vi "Exp2.vi"() -> ()   [LabVIEW 2018]
uses:
  <vilib>/Platform/TimedLoop/XDataNode/timing_clust.ctl
  <vilib>/Platform/TimedLoop/XDataNode/nitl_modes.ctl
  <vilib>/Platform/TimedLoop/XDataNode/wakeup.ctl
  <vilib>/MakerHub/LINX/Public/Peripherals/Analog/Analog Read 1 Chan.vi
  <vilib>/MakerHub/LINX/Public/Peripherals/PWM/PWM Set Duty Cycle 1 Chan.vi
  <vilib>/MakerHub/LINX/Public/Peripherals/Analog/Analog Read N Chans.vi
  <vilib>/MakerHub/LINX/Private/Local IO/LinxAnalogRead.vi
  <vilib>/MakerHub/LINX/Public/Utilities/Check Channel.vi
  <vilib>/MakerHub/LINX/Public/Utilities/Open Serial.vi
  <vilib>/MakerHub/LINX/Private/Utilties/Generate Error.vi
  <vilib>/MakerHub/LINX/Public/Peripherals/PWM/PWM Set Duty Cycle N Chans.vi
  <vilib>/platform/TimedLoop/XDataNode/XDataNode.xnode
  <vilib>/MakerHub/LINX/LMH-LINX.lvlib
  <vilib>/Platform/TimedLoop/XDataNode/XDNodeRunTimeDep.lvlib
panel:
  out "T0":dbl
  in  "Tab Control":enum32{"Monitoring", "TDTC Model"}(tab)
  out "Temperature":cluster{dbl, "output":dbl}(graph)={31.0, "output"=73.73046875}
  out "Overrun":bool
  in  "Serial Port":refnum<visa-resource-name>="COM4"
  in  "Duty Cycle (0-100)":dbl min=0.0 max=1.0 step=0.1
  out "Period":i64
  in  "Kss":dbl=1.1
  in  "Theta":dbl=9.49
  in  "Tau":dbl=232.06
  in  "Stop Button":bool
  # "TDTC Model Parameters"
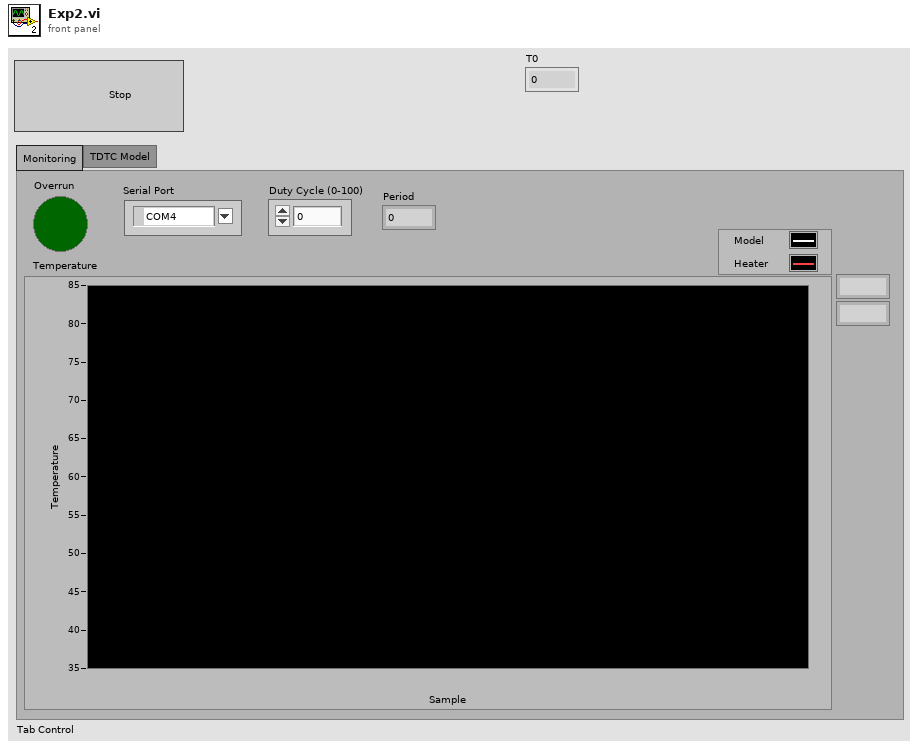
[diagram p1: front panel]
types:
  T1 = enum16{"open", "replace", "create", "open or create", "replace or create", "replace or create with confirmation"}
  T2 = typedef "XDNodeRunTimeDep.lvlib/timing_clust.ctl" = cluster{"Expected End [f-1]":u64, "Actual End [f-1]":u64, "Finished Late? [f-1]":bool, "Expected End [i-1]":u64, "Actual End [i-1]":u64, "Finished Late? [i-1]":bool, "Expected Start [i]":u64, "Actual Start [i]":u64, "Expected Start [f]":u64, "Actual Start [f]":u64, "Source Name":string, "Structure Name":string, "Period":i64, "Deadline":i64, "Offset":i64, "Start":i64, "Priority":i32, "Timeout":i32, "Mode":T3, "Wakeup Reason":T4, "Error":errorcluster, "Source Type":string, "Secondary Source Type":string, "Global End Time":u64, "Global Start Time":u64, "Frame Duration":u64, "Iteration Duration":u64, "Assigned CPU":i32, "I/O Scan Engine Mode":u32}
  T3 = typedef "XDNodeRunTimeDep.lvlib/nitl_modes.ctl" = enum32{"No Change", "Process missed periods, maintain original phase", "Discard missed periods, maintain original phase", "Process missed periods, ignore original phase", "Discard missed periods, ignore original phase"}
  T4 = typedef "XDNodeRunTimeDep.lvlib/wakeup.ctl" = enum32{"Normal", "Aborted", "Asynchronous wakeup", "Timing source error", "Timed loop error", "Timeout"}
  T5 = typedef "LMH-LINX.lvlib/LINX Ref.ctl" = cluster{"IO":T6, "Interface":T7, "LINX Device Config":T8}
  T6 = typedef "LMH-LINX.lvlib/Platform.ctl" = enum16{"Remote", "Local"}
  T7 = typedef "LMH-LINX.lvlib/Interface.ctl" = enum16{"Serial", "TCP"}
  T8 = typedef "LMH-LINX.lvlib/Device.lvlib/LINX Device Config.ctl" = cluster{"Interface":T7, "COM Port":refnum<visa-resource-name>, "TCP Configuration":T9, "Device Family":u8, "Device ID":u8, "Device Name":string, "TCP Ref":refnum<k5>, "Channels":T10}
  T9 = typedef "LMH-LINX.lvlib/Device.lvlib/TCP Config.ctl" = cluster{"IP Address":string, "Port":u16}
  T10 = typedef "LMH-LINX.lvlib/Channels.ctl" = cluster{"DI":u8[], "DO":u8[], "AI":u8[], "AO":u8[], "PWM":u8[], "QE":u8[], "UART":u8[], "I2C 2":u8[], "SPI":u8[], "CAN":u8[], "Servo":u8[], "AI Ref (V)":dbl, "AI Resolution (Bits)":u8, "AO Ref (V)":dbl, "AO Resolution (Bits)":u8}
  T11 = enum16{"big-endian, network order", "native, host order", "little-endian"}
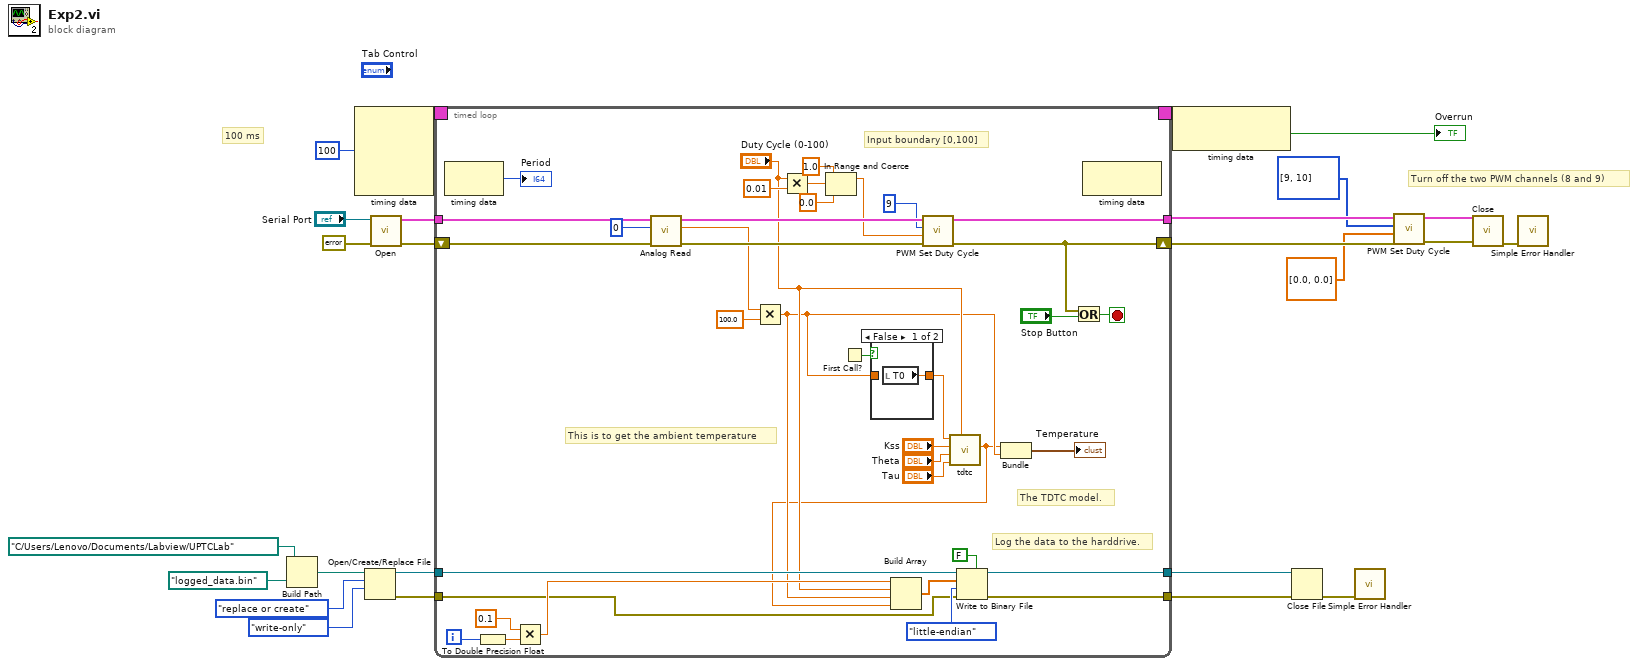
[diagram p0: block diagram]
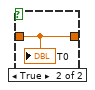
[diagram p2: hidden frame]
diagram:
  # "100 ms"
  # "Turn off the two PWM channels (8 and 9)"
  n1 = Build Path(base path=path "C:/Users/Lenovo/Documents/Labview/UPTCLab", name or relative path=path "logged_data.bin" ("default name")) -> (appended path=w3:path)
  n2 = node-c288(i64 100 ("Period")) -> (w20:T2)  [unwired: 3 in]
  n3 = Open/Create/Replace File(file path (use dialog)=w3, operation (0:open)=T1."replace or create", access (0:read/write)=enum16{"read/write", "read-only", "write-only"}."write-only") -> (refnum out=w7:refnum<file>, error out=w1:errorcluster)  [unwired: 3 in, 1 out]
  n4 = call-poly <vilib>:"Open.vi"("Error In"=errorcluster {"status"=FALSE, "code"=0, "source"=""}, "Serial Port"="Serial Port") -> ("Error Out"=w24:errorcluster, "LINX Resource"=w25:T5)  [unwired: 7 in, 1 out]
  n5 = timed-loop {
    tunnel: w25 -> [w61]
    tunnel: [w56] -> w16
    shift-right: [w55] -> w15
    shift-left: w24 -> [w60]
    timing: w20 -> [_]
    timing-out: [_] -> w19
    tunnel: w7 -> [w45]
    tunnel: [w38] -> w5
    tunnel: [w37] -> w4
    tunnel: w1 -> [w26]
    i -> [w44]
    stop <- w63 stop-if-true
    # "Log the data to the harddrive."
    # "The TDTC model."
    # "Input boundary [0,100]"
    # "This is to get the ambient temperature"
    n6 = node-c288() -> (→"Period":i64)  [unwired: 1 in]
    n7 = To Double Precision Float(number=w44) -> (double precision float=w43:dbl)
    n8 = Multiply(x=0.1, y=w43) -> (x*y=w36:dbl)
    n9 = call-poly <vilib>:"Analog Read.vi"("Error In"=w60, "Analog Channel"=u8 0, "LINX Resource"=w61) -> ("Error Out"=w57:errorcluster, "Voltage"=w53:dbl, "LINX Resource"=w58:T5)  [unwired: 5 in, 1 out]
    n10 = Multiply(x=w53, y=100.0) -> (x*y=w29:dbl)
    n11 = Multiply(x="Duty Cycle (0-100)", y=0.01) -> (x*y=w49:dbl)
    n12 = In Range and Coerce(upper limit=1.0, x=w49, lower limit=0.0) -> (coerced(x)=w48:dbl)  [unwired: 1 out]
    n13 = First Call?() -> (First Call?: T/F=w30:bool)
    n14 = case shown="False" w30 {
      tunnel: w29 -> [_ w65]
      tunnel: [w64 w65] -> w28
      frame False {
        n15 = local read "T0"() -> (w64:dbl)
      }
      frame True {
        "T0" <- w65
      }
    }
    n16 = call-poly <vilib>:"PWM Set Duty Cycle.vi"("Error In"=w57, "Duty Cycle (0-1)"=w48, "PWM Channel"=u8 9, "LINX Resource"=w58) -> ("Error Out"=w55:errorcluster, "LINX Resource"=w56:T5)  [unwired: 6 in]
    n17 = call "tdtc.vi"("input"="Duty Cycle (0-100)", "Tau"="Tau", "Theta"="Theta", "Kss"="Kss", "T0"=w28) -> ("output"=w27:dbl)  [unwired: 6 in]
    n18 = Build Array(w36, "Duty Cycle (0-100)", w29, w27) -> (w41:dbl[])
    n19 = Write to Binary File(file (use dialog)=w45, data=w41, error in=w26, 5:FALSE ("prepend array or string size? (T)"), 9:T11."little-endian" ("byte order (0:big-endian, network order)")) -> (refnum out=w38:refnum<file>, error out=w37:errorcluster)  [unwired: 1 in, 1 out]
    n20 = Bundle("output"=w27, w29) -> (→"Temperature":cluster{"output":dbl, dbl})  [unwired: 1 in]
    n21 = Or(x=w55, y="Stop Button") -> (x .or. y?=w63:bool)
    n22 = node-c288() -> ()  [unwired: 1 in, 1 out]
  }
  n23 = node-c288(w19) -> (→"Overrun":bool)
  n24 = Close File(refnum=w5, error in=w4) -> (error out=w6:errorcluster)  [unwired: 1 out]
  n25 = call <vilib>:"Simple Error Handler.vi"("error in (no error)"=w6) -> ()  [unwired: 4 in, 5 out]
  n26 = call-poly <vilib>:"PWM Set Duty Cycle.vi"("Error In"=w15, "Duty Cycles"=dbl[] [0.0, 0.0], "PWM Channels"=u8[] [9, 10], "LINX Resource"=w16) -> ("Error Out"=w14:errorcluster, "LINX Resource"=w17:T5)  [unwired: 6 in]
  n27 = call <vilib>:"Close.vi"("Error In"=w14, "LINX Resource"=w17) -> ("Error Out"=w22:errorcluster)  [unwired: 9 in]
  n28 = call <vilib>:"Simple Error Handler.vi"("error in (no error)"=w22) -> ()  [unwired: 4 in, 5 out]
